vi "ContextHelp_StartPopUpTask1.vi"(0 "PopUpTaskEvent":T1, 1 "OpenState":bool, 5 "error in (no error)":errorcluster, 6 "Actio(GetStatus)n":T2(ring)=enum."GetStatus") -> (14 "PopUpTaskEventOut":T1, 15 "Open":bool, 19 "error out":errorcluster)   [LabVIEW 2014]
uses:
  <resource>/Framework/Providers/Open_GDS/UML/ContextHelp/ContextHelp_EventType.ctl
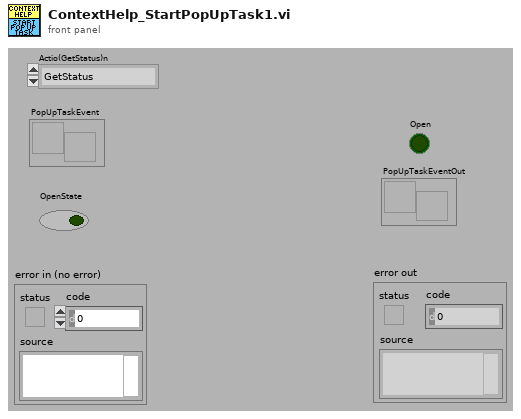
[diagram p1: front panel]
types:
  T1 = typedef "ContextHelp_EventType.ctl" = refnum<user-event>
  T2 = enum16{"SetPopUpEventTask", "GetStatus", "SetOpenState"}
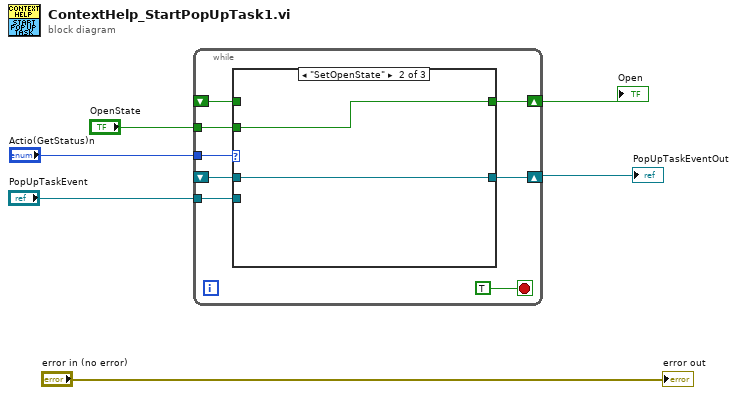
[diagram p0: block diagram]
diagram:
  n1 = while {
    tunnel: "Actio(GetStatus)n" -> [w14]
    shift-right: [w12] -> w4
    shift-left: _ -> [w13]
    tunnel: "OpenState" -> [w11]
    shift-right: [w10] -> w1
    shift-left: _ -> [w8]
    tunnel: "PopUpTaskEvent" -> [w9]
    stop <- TRUE stop-if-true
    n2 = case shown="\"SetOpenState\"" w14 {
      tunnel: w13 -> [w16 _ w20]
      tunnel: [w16 w18 w20] -> w12
      tunnel: w11 -> [_ w18 _]
      tunnel: [w15 w17 w19] -> w10
      tunnel: w9 -> [w15 _ _]
      tunnel: w8 -> [_ w17 w19]
      frame "SetPopUpEventTask", Default {
      }
      frame "SetOpenState" {
      }
      frame "GetStatus" {
      }
    }
  }
  "Open" <- w4
  "PopUpTaskEventOut" <- w1
  "error out" <- "error in (no error)"
